vi "Config System Actors.vi"(7 "Config Parameters":T1, 8 "error in (no error)":errorcluster, 10 "Root Actor In":refnum<class "Root Actor.lvclass">, 11 "System Modules Factory in":refnum<class "System Modules Factory.lvclass">) -> (0 "error out":errorcluster, 2 "Root Actor Out":refnum<class "Root Actor.lvclass">, 3 "System Modules Factory out":refnum<class "System Modules Factory.lvclass">)   [LabVIEW 2019, in "System Modules Factory.lvclass"]
uses:
  System Modules Factory.lvclass
  Actor/Root Actor/Root Actor.lvclass
  C:/Users/iio/Desktop/NTHU Brain Center/General Library/Ancestor Class/Actor/System Actor/System Actor.lvclass
  Type Def/Config Parameters.ctl
  Messenger/Mail Strategy/Mail Strategy.lvclass
  Actor/System Actor/System Actor.lvclass
  Actor/System Actor/System Actor.lvclass/System Actor.ctl
  Actor/Root Actor/Root Actor.lvclass/Root Actor.ctl
  Actor/System Actor/Public Data/Write Self Messenger Location.vi
  Actor/System Actor/Public Data/Write Stop Notifier.vi
  Actor/Root Actor/Protected Data/Accept VI Refs.vi
  Actor/Root Actor/Public Data/Write Modules Stop Notifier.vi
  General Parent Class/Enumeration Tree Queue Mailman/Enumeration Tree Queue Mailman.lvclass
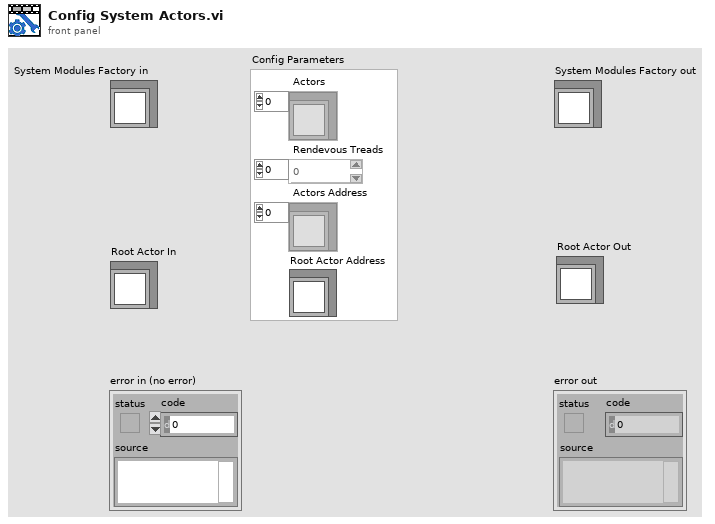
[diagram p1: front panel]
types:
  T1 = typedef "Config Parameters.ctl" = cluster{"Actors":refnum<class "System Actor.lvclass">[], "Rendevous Treads":i32[], "Actors Address":refnum<class "Mail Strategy.lvclass">[], "Root Actor Address":refnum<class "Mail Strategy.lvclass">}
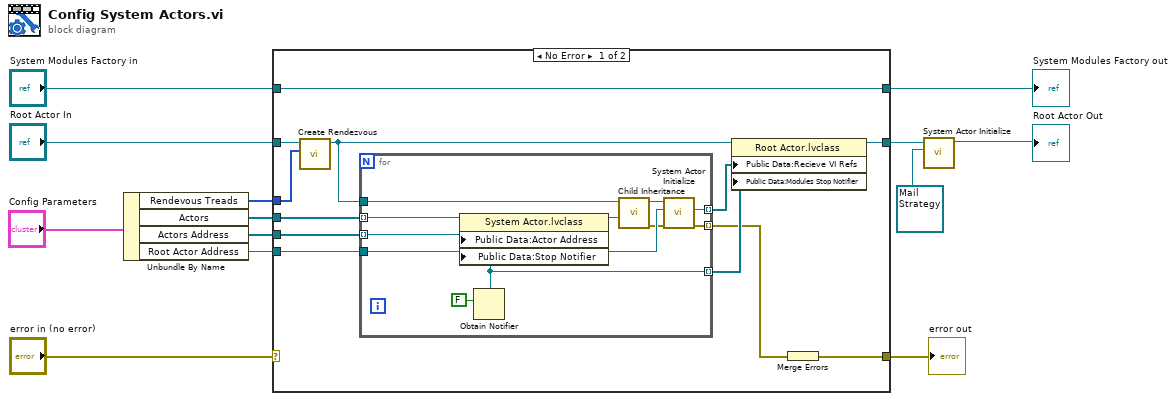
[diagram p0: block diagram]
diagram:
  n1 = Unbundle By Name("Config Parameters") -> ("Rendevous Treads"=w5:i32[], "Actors"=w7:refnum<class "System Actor.lvclass">[], "Actors Address"=w6:refnum<class "Mail Strategy.lvclass">[], "Root Actor Address"=w4:refnum<class "Mail Strategy.lvclass">)
  n2 = case shown="No Error" "error in (no error)" {
    selector: "error in (no error)" -> [_ w39]
    tunnel: [w14 w39] -> w12
    tunnel: [w25 w38] -> w10
    tunnel: "System Modules Factory in" -> [w25 w38]
    tunnel: "Root Actor In" -> [w23 w37]
    tunnel: w7 -> [w24 _]
    tunnel: [w21 w37] -> w3
    tunnel: w6 -> [w20 _]
    tunnel: w5 -> [w19 _]
    tunnel: w4 -> [w18 _]
    frame No Error {
      n3 = call "Create Rendezvous.vi"("Treads"=w19, "Actor In"=w23) -> ("Actor Out"=w22:refnum<class "Root Actor.lvclass">)  [unwired: 8 in, 1 out]
      n4 = for {
        tunnel: w22 -> [w36]
        tunnel: w24 -> [w34] mode=indexing
        tunnel: [w35] -> w17 mode=indexing
        tunnel: w20 -> [w33] mode=indexing
        tunnel: w18 -> [w32]
        tunnel: [w31] -> w16 mode=indexing
        tunnel: [w26] -> w15 mode=indexing
        n5 = Obtain Notifier(notification data type=FALSE) -> (notifier out=w31:refnum<notifier>)  [unwired: 3 in, 2 out]
        n6 = property class="System Actor.lvclass"(reference=w34, "Public Data:Actor Address"=w33, "Public Data:Stop Notifier"=w31) -> (reference out=w28:refnum<class "System Actor.lvclass">)  [unwired: 1 in, 1 out]
        n7 = call "Child Inheritance.vi"("Child In"=w28, "Ancestor In"=w36) -> ("error out"=w29:errorcluster, "Child Out"=w30:refnum<class "System Actor.lvclass">)  [unwired: 8 in]
        n8 = call-dynamic "System Actor Initialize.vi"("error in (no error)"=w29, "Root Actor Address"=w32, "System Actor in"=w30) -> ("error out"=w26:errorcluster, "VI Refnum"=w35:refnum<vi>)  [unwired: 6 in, 1 out]
      }
      n9 = property class="Root Actor.lvclass"(reference=w22, "Public Data:Recieve VI Refs"=w17, "Public Data:Modules Stop Notifier"=w16) -> (reference out=w21:refnum<class "Root Actor.lvclass">)  [unwired: 1 in, 1 out]
      n10 = Merge Errors(w15) -> (w14:errorcluster)
    }
    frame Error {
    }
  }
  "error out" <- w12
  "System Modules Factory out" <- w10
  n11 = call-dynamic "System Actor Initialize.vi"("Root Actor Address"=refnum<class "Mail Strategy.lvclass"> refnum, "System Actor in"=w3) -> ("System Actor out"=→"Root Actor Out":refnum<class "Root Actor.lvclass">)  [unwired: 7 in, 2 out]
